vi "GetVisaRes.vi"(8 "error in (no error)":errorcluster caption="entrée d'erreur (pas d'erreur)", 11 "Device en entrée":refnum<class "BaseDevice.lvclass"> caption="DNL_LabVIEW Object in") -> (0 "error out":errorcluster caption="sortie d'erreur", 2 "ResVISA":refnum<visa-resource-name>, 3 "Device en sortie":refnum<class "BaseDevice.lvclass"> caption="DNL_LabVIEW Object out")   [LabVIEW 2019, in "BaseDevice.lvclass"]
uses:
  BaseDevice.lvclass
  BaseDevice.lvclass/BaseDevice.ctl
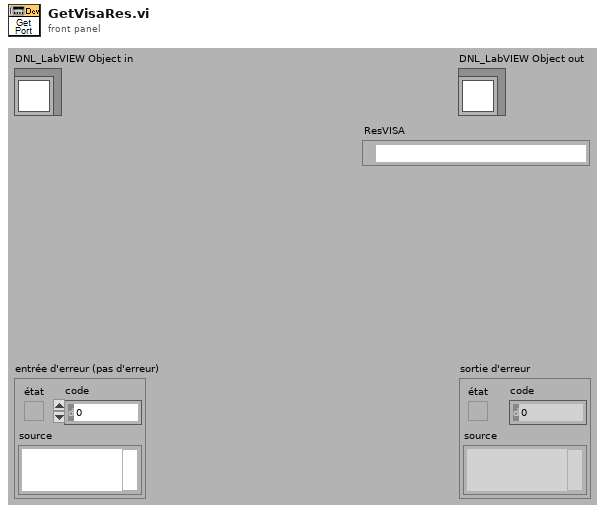
[diagram p1: front panel]
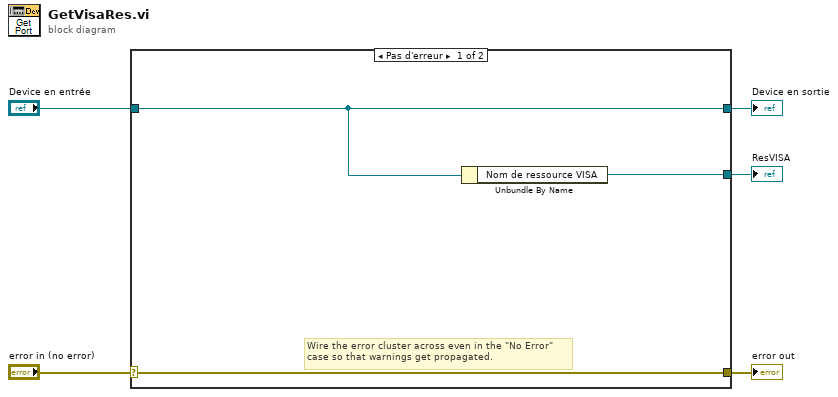
[diagram p0: block diagram]
diagram:
  n1 = case shown="Pas d'erreur" "error in (no error)" {
    selector: "error in (no error)" -> [w8 w10]
    tunnel: [w8 w10] -> w4
    tunnel: [w7 w9] -> w2
    tunnel: "Device en entrée" -> [w7 w9]
    tunnel: [w6 _] -> w1
    frame No Error {
      # "Wire the error cluster across even in the \"No Error\"\ncase so that warnings get propagated."
      n2 = Unbundle By Name(w7) -> ("Nom de ressource VISA"=w6:refnum<visa-resource-name>)
    }
    frame Error {
    }
  }
  "error out" <- w4
  "Device en sortie" <- w2
  "ResVISA" <- w1
